vi "read_settings_file.vi"(8 "error in (no error)":errorcluster, 10 "settings name":string, 11 "GenericPlugin in":refnum<class "StringGeneratorAK110125StimServerCmd.lvclass">) -> (0 "error out":errorcluster, 1 "cancelled?":bool, 2 "settings cluster out":variant, 3 "GenericPlugin out":refnum<class "StringGeneratorAK110125StimServerCmd.lvclass">, 4 "settings name":string)   [LabVIEW 2010, in "StringGeneratorAK110125StimServerCmd.lvclass"]
uses:
  StringGeneratorAK110125StimServerCmd.lvclass
  GenericStringGenerator/GenericStringGenerator/GenericStringGenerator.lvclass
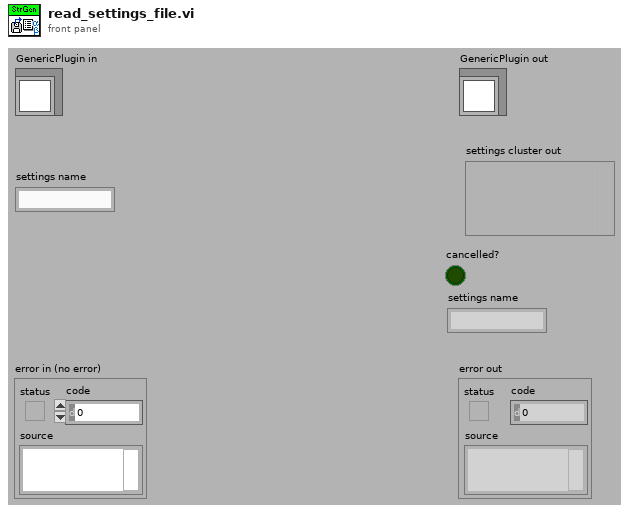
[diagram p1: front panel]
types:
  T1 = cluster{"stimulus IDs with spaces":string, "stimulus":string, "blank time (s)":string, "randomize":bool, "user sequence":bool}
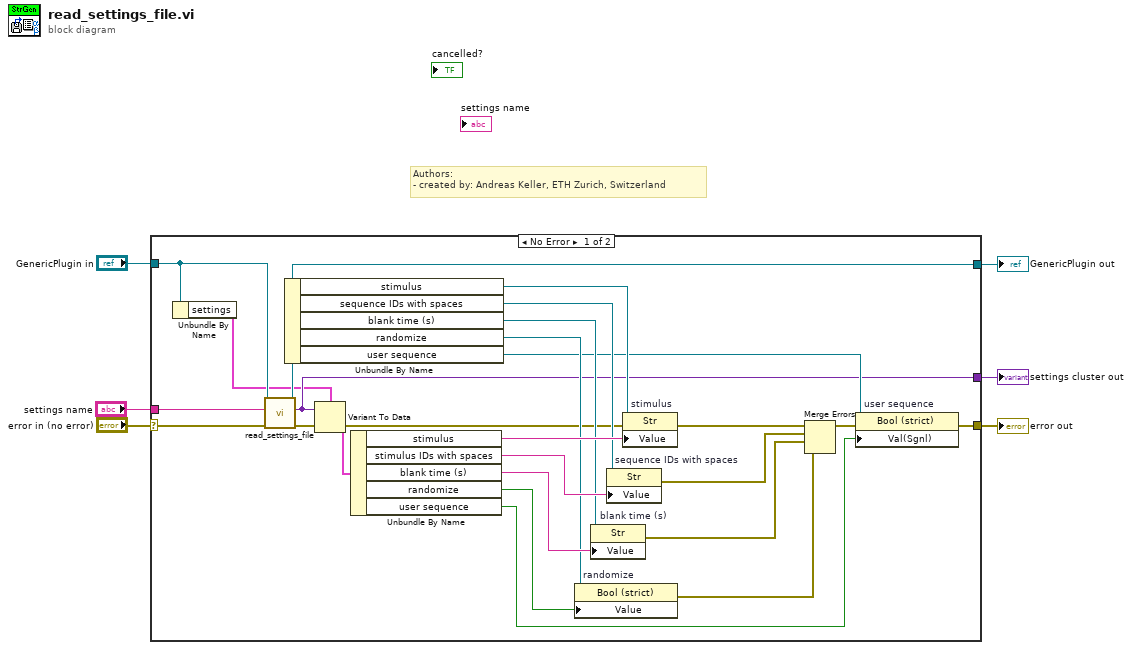
[diagram p0: block diagram]
diagram:
  # "Authors: \n- created by: Andreas Keller, ETH Zurich, Switzerland"
  n1 = case shown="No Error" "error in (no error)" {
    selector: "error in (no error)" -> [w30 w31]
    tunnel: [w10 w31] -> w5
    tunnel: "settings name" -> [w29 _]
    tunnel: "GenericPlugin in" -> [w28 w32]
    tunnel: [w8 _] -> w2
    tunnel: [w26 w32] -> w1
    frame No Error {
      n2 = Unbundle By Name(w28) -> ("settings"=w7:T1)
      n3 = call-parent "read_settings_file.vi"("error in (no error)"=w30, "settings name"=w29, "GenericComponent in"=w28) -> ("error out"=w27:errorcluster, "settings cluster out"=w8:variant, "GenericComponent out"=w26:refnum<class "StringGeneratorAK110125StimServerCmd.lvclass">)  [unwired: 4 in, 2 out]
      n4 = Unbundle By Name(w26) -> ("stimulus"=w24:refnum<vi>, "sequence IDs with spaces"=w19:refnum<vi>, "blank time (s)"=w20:refnum<vi>, "randomize"=w18:refnum<vi>, "user sequence"=w17:refnum<vi>)
      n5 = Variant To Data(error in=w27, Variant=w8, type=w7) -> (error out=w11:errorcluster, data=w25:T1)
      n6 = Unbundle By Name(w25) -> ("stimulus"=w23:string, "stimulus IDs with spaces"=w22:string, "blank time (s)"=w21:string, "randomize"=w16:bool, "user sequence"=w9:bool)
      n7 = property on="randomize" class="Bool (strict)"(reference=w18, "Value"=w16) -> (error out=w13:errorcluster)  [unwired: 1 in, 1 out]
      n8 = property on="blank time (s)" class="Str"(reference=w20, "Value"=w21) -> (error out=w14:errorcluster)  [unwired: 1 in, 1 out]
      n9 = property on="sequence IDs with spaces" class="Str"(reference=w19, "Value"=w22) -> (error out=w15:errorcluster)  [unwired: 1 in, 1 out]
      n10 = property on="stimulus" class="Str"(reference=w24, error in=w11, "Value"=w23) -> ()  [unwired: 2 out]
      n11 = Merge Errors(w11, w15, w14, w13) -> (w12:errorcluster)
      n12 = property on="user sequence" class="Bool (strict)"(reference=w17, error in=w12, "Val(Sgnl)"=w9) -> (error out=w10:errorcluster)  [unwired: 1 out]
    }
    frame Error {
    }
  }
  "error out" <- w5
  "GenericPlugin out" <- w1
  "settings cluster out" <- w2
